vi "Connect.vi"(8 "error in (no error)":errorcluster) -> (0 "error out":errorcluster, 2 "controller":refnum<k24>, 3 "controllers":refnum<k24>[](array[refnum]))   [LabVIEW 2013]
uses:
  C:/GEECS/Developers Version/source/Device Driver/AerotechStage/Sample Vis/Bin/Aerotech.Ensemble.dll
  Bin/Aerotech.Ensemble.dll
  C:/GEECS/Developers Version/source/Device Driver/AerotechStage/Sample Vis/Bin/Aerotech.Ensemble.LabVIEW.dll
  Bin/Aerotech.Ensemble.LabVIEW.dll
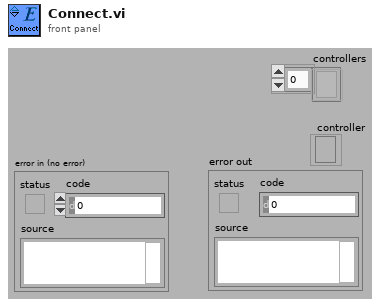
[diagram p1: front panel]
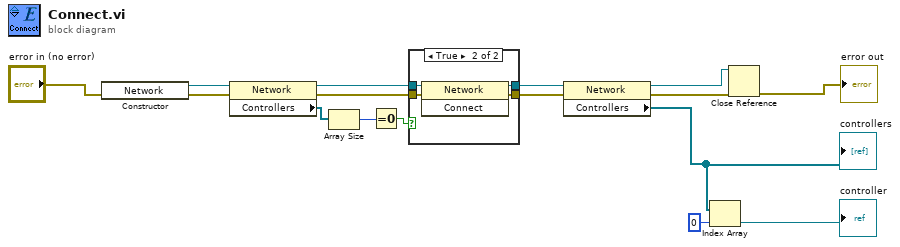
[diagram p0: block diagram]
diagram:
  n1 = constructor class="Network"(error in="error in (no error)") -> (reference out=w6:refnum<k24>, error out=w7:errorcluster)  [unwired: 2 in, 1 out]
  n2 = property class="Network"(reference=w6, error in=w7) -> (reference out=w5:refnum<k24>, error out=w11:errorcluster, "Controllers"=w12:refnum<k24>[])
  n3 = Array Size(array=w12) -> (size(s)=w10:i32)
  n4 = Equal To 0?(x=w10) -> (x = 0?=w9:bool)
  n5 = case shown="True" w9 {
    tunnel: [w18 w22] -> w16
    tunnel: w11 -> [w18 w21]
    tunnel: w5 -> [w17 w20]
    tunnel: [w17 w19] -> w4
    frame False {
    }
    frame True {
      n6 = invoke class="Network" method="Connect"(reference=w20, error in=w21) -> (reference out=w19:refnum<k24>, error out=w22:errorcluster)  [unwired: 1 in, 1 out]
    }
  }
  n7 = property class="Network"(reference=w4, error in=w16) -> (reference out=w1:refnum<k24>, error out=w3:errorcluster, "Controllers"=w15:refnum<k24>[])
  "controllers" <- w15
  n8 = Index Array(array=w15, index=0) -> (element=→"controller":refnum<k24>)
  n9 = Close Reference(reference=w1, error in (no error)=w3) -> (error out=→"error out":errorcluster)
